vi "CovarianceToGraph.vi"(10 "Mu":T1, 11 "covariance matrix":T1=[[1.0, 0.0], [0.0, 1.0]]) -> (3 "XY Graph":cluster{cdb[], cdb[]})   [LabVIEW 2017]
uses:
  <vilib>/Analysis/Matrix/Datatypes/RealMatrix.ctl
  <vilib>/Analysis/baseanly.llb/Complex A x B.vi
  <vilib>/Analysis/baseanly.llb/Complex A x Vector.vi
  <vilib>/Analysis/7linalg.llb/Real Eigenvalues and Vectors.vi
  <vilib>/Analysis/Matrix/Numeric/Conversions/Matrix To Array - RM.vi
  <vilib>/Analysis/NI_AALPro.lvlib
  <vilib>/Analysis/NI_AALBase.lvlib
  <vilib>/Analysis/Matrix/NI_Matrix.lvlib
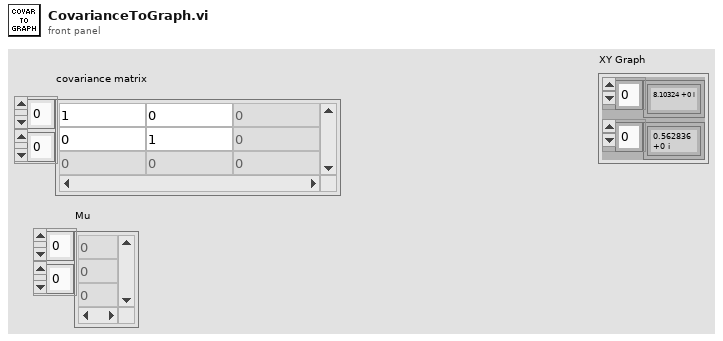
[diagram p1: front panel]
types:
  T1 = typedef "NI_Matrix.lvlib/RealMatrix.ctl" = dbl[][]
  T2 = typedef "NI_Matrix.lvlib/ComplexMatrix.ctl" = cdb[][]
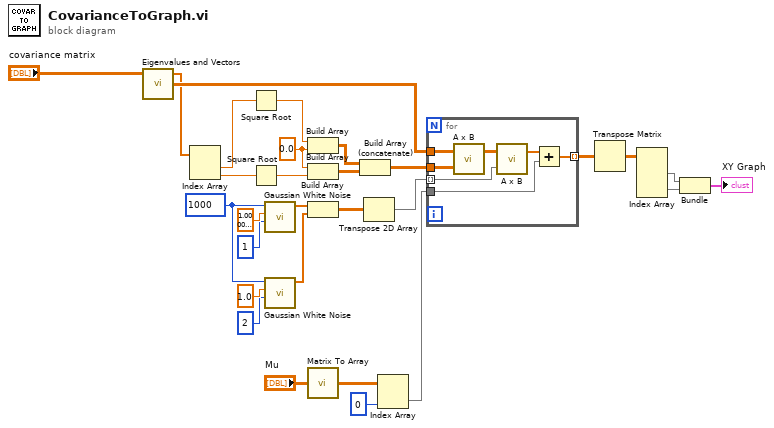
[diagram p0: block diagram]
diagram:
  w12 = 1000 ("samples")
  w27 = 0.0 ("element")
  n1 = call-poly <vilib>:"Eigenvalues and Vectors.vi"("Input Matrix"="covariance matrix") -> ("Eigenvectors"=w18:T2, "Eigenvalues"=w17:cdb[])  [unwired: 2 in, 1 out]
  n2 = Index Array(array=w17) -> (element #1=w22:cdb, element #2=w20:cdb)  [unwired: 2 in]
  n3 = Square Root(x=w22) -> (sqrt(x)=w21:cdb)
  n4 = Square Root(x=w20) -> (sqrt(x)=w19:cdb)
  n5 = call <vilib>:"Gaussian White Noise.vi"("seed"=1, "standard deviation"=1.0000000000000002, "samples"=w12) -> ("Gaussian noise pattern"=w11:dbl[])  [unwired: 7 in, 1 out]
  n6 = call <vilib>:"Gaussian White Noise.vi"("seed"=2, "standard deviation"=1.0, "samples"=w12) -> ("Gaussian noise pattern"=w10:dbl[])  [unwired: 7 in, 1 out]
  n7 = Build Array(w21, w27) -> (w28:T2)
  n8 = Build Array(w27, w19) -> (w29:T2)
  n9 = Build Array(w11, w10) -> (w9:dbl[][])
  n10 = call-poly <vilib>:"Matrix To Array.vi"("Real Matrix"="Mu") -> ("Real 2D Array"=w4:dbl[][])
  n11 = Build Array (concatenate)(w28, w29) -> (w15:T2)
  n12 = Transpose 2D Array(2D array=w9) -> (transposed array=w8:dbl[][])
  n13 = Index Array(array=w4, index (col)=0 ("disabled index (col)")) -> (element=w1:dbl[])  [unwired: 1 in]
  n14 = for {
    tunnel: w8 -> [w36] mode=indexing
    tunnel: [w31] -> w24 mode=indexing
    tunnel: w15 -> [w33]
    tunnel: w18 -> [w34]
    tunnel: w1 -> [w30]
    n15 = call-poly <vilib>:"A x B.vi"("B"=w33, "A"=w34) -> ("A x B"=w35:T2)  [unwired: 1 out]
    n16 = call-poly <vilib>:"A x B.vi"("Vector"=w36, "A"=w35) -> ("A x Vector"=w32:cdb[])  [unwired: 1 out]
    n17 = Add(x=w32, y=w30) -> (x+y=w31:cdb[])
  }
  n18 = Transpose Matrix(1:w24) -> (0:w26:cdb[][])
  n19 = Index Array(array=w26) -> (element #1=w25:cdb[], element #2=w23:cdb[])  [unwired: 4 in]
  n20 = Bundle(w25, w23) -> (→"XY Graph":cluster{cdb[], cdb[]})  [unwired: 1 in]
